vi "VNA_ReadConf.vi"(8 "error in":errorcluster, 10 "VNAClusterIn":T3={"Value"=0.0, "GUI Data Cluster"={"S11"=FALSE, "S21"=FALSE, "S12"=FALSE, "S22"=FALSE, "S11Meas"=enum."Log-magnitude (dB)", "S21Meas"=enum."Log-magnitude (dB)", "S12Meas"=enum."Log-magnitude (dB)", "S22Meas"=enum."Log-magnitude (dB)"}, "Timing"={"Last Operation"=0.0, "Stop @ T/B"=FALSE, "Last Temp"=0.0, "Last Mag"=0.0, "Ramp Param"={"End T (K)"=0.0, "Delta T (K)"=0.0, "End B (T)"=0.0, "Delta B (T)"=0.0}, "LastOp?"=FALSE, "FirstOp?"=FALSE}, "Measurements"=[], "Hardware"={"VNA TCP Con"=refnum, "VNA TCP Port"=5025, "Global T VAR"="", "Global B VAR"=""}, "Operation"={"Operation Mode"=enum."Logging", "Log Folder"=path "", "Measure Mode"=enum."Deltat"}}, 11 "GeneralClusterIn":T1) -> (0 "error out":errorcluster, 2 "VNAClusterOut":T3={"Value"=0.0, "GUI Data Cluster"={"S11"=FALSE, "S21"=FALSE, "S12"=FALSE, "S22"=FALSE, "S11Meas"=enum."Log-magnitude (dB)", "S21Meas"=enum."Log-magnitude (dB)", "S12Meas"=enum."Log-magnitude (dB)", "S22Meas"=enum."Log-magnitude (dB)"}, "Timing"={"Last Operation"=0.0, "Stop @ T/B"=FALSE, "Last Temp"=0.0, "Last Mag"=0.0, "Ramp Param"={"End T (K)"=0.0, "Delta T (K)"=0.0, "End B (T)"=0.0, "Delta B (T)"=0.0}, "LastOp?"=FALSE, "FirstOp?"=FALSE}, "Measurements"=[], "Hardware"={"VNA TCP Con"=refnum, "VNA TCP Port"=5025, "Global T VAR"="", "Global B VAR"=""}, "Operation"={"Operation Mode"=enum."Logging", "Log Folder"=path "", "Measure Mode"=enum."Deltat"}}, 3 "GeneralClusterOut":T1)   [LabVIEW 2021]
uses:
  Library/TerminalDef.ctl
  <vilib>/Utility/config.llb/Config Data RefNum.ctl
  Data_Cluster.ctl
  Measurement_Cluster.ctl
  Mode_Enum.ctl
  Library/LibDan.lvlib
  <vilib>/Utility/config.llb/NI_LVConfig.lvlib
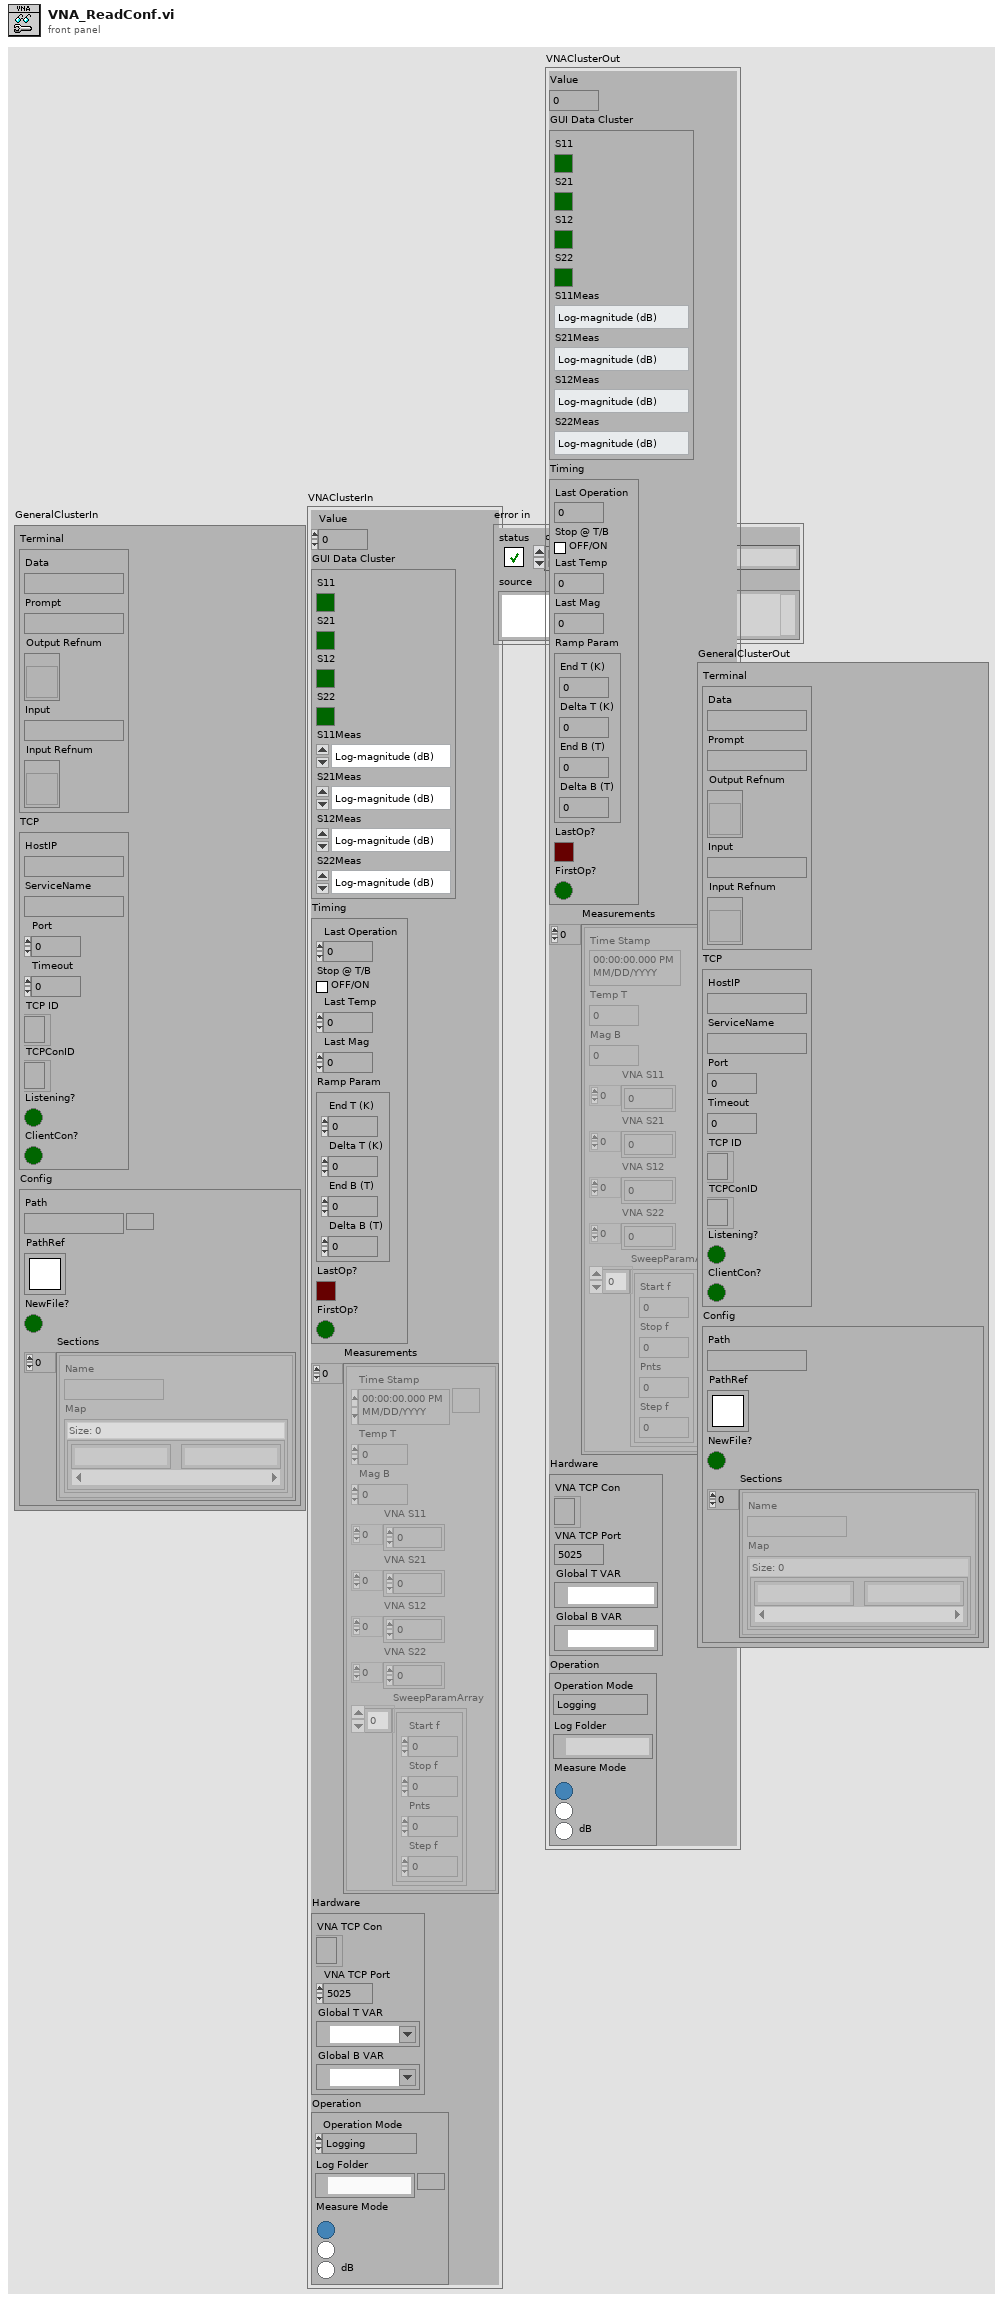
[diagram p1: front panel]
types:
  T1 = typedef "LibDan.lvlib/TerminalDef.ctl" = cluster{"Terminal":cluster{"Data":string, "Prompt":string, "Output Refnum":refnum<vi>, "Input":string, "Input Refnum":refnum<vi>}, "TCP":cluster{"HostIP":string, "ServiceName":string, "Port":u16, "Timeout":i32, "TCP ID":refnum<k5>, "TCPConID":refnum<k5>, "Listening?":bool, "ClientCon?":bool}, "Config":cluster{"Path":path, "PathRef":T2, "NewFile?":bool, "Sections":cluster{"Name":string, "Map":map{string, string}}[]}}
  T2 = typedef "NI_LVConfig.lvlib/Config Data RefNum.ctl" = refnum<k1>
  T3 = typedef "Data_Cluster.ctl" = cluster{"Value":dbl, "GUI Data Cluster":cluster{"S11":bool, "S21":bool, "S12":bool, "S22":bool, "S11Meas":enum16{"Log-magnitude (dB)", "Linear magnitude", "Phase (deg)", "Time Domain", "Real", "Imaginary", "Group Delay", "Polarlinear"}, "S21Meas":enum16{"Log-magnitude (dB)", "Linear magnitude", "Phase (deg)", "Time Domain", "Real", "Imaginary", "Group Delay", "Polarlinear"}, "S12Meas":enum16{"Log-magnitude (dB)", "Linear magnitude", "Phase (deg)", "Time Domain", "Real", "Imaginary", "Group Delay", "Polarlinear"}, "S22Meas":enum16{"Log-magnitude (dB)", "Linear magnitude", "Phase (deg)", "Time Domain", "Real", "Imaginary", "Group Delay", "Polarlinear"}}, "Timing":cluster{"Last Operation":dbl, "Stop @ T/B":bool, "Last Temp":dbl, "Last Mag":dbl, "Ramp Param":cluster{"End T (K)":dbl, "Delta T (K)":dbl, "End B (T)":dbl, "Delta B (T)":dbl}, "LastOp?":bool, "FirstOp?":bool}, "Measurements":T4[], "Hardware":cluster{"VNA TCP Con":refnum<k5>, "VNA TCP Port":i32, "Global T VAR":refnum<k21>, "Global B VAR":refnum<k21>}, "Operation":cluster{"Operation Mode":T5, "Log Folder":path, "Measure Mode":enum32{"Deltat", "DeltaT", "dB"}}}
  T4 = typedef "Measurement_Cluster.ctl" = cluster{"Time Stamp":timestamp, "Temp T":dbl, "Mag B":dbl, "VNA S11":dbl[], "VNA S21":dbl[], "VNA S12":dbl[], "VNA S22":dbl[], "SweepParamArray":cluster{"Start f":dbl, "Stop f":dbl, "Pnts":i32, "Step f":dbl}[]}
  T5 = typedef "Mode_Enum.ctl" = enum16{"Logging", "Idle-Off", "Idle"}
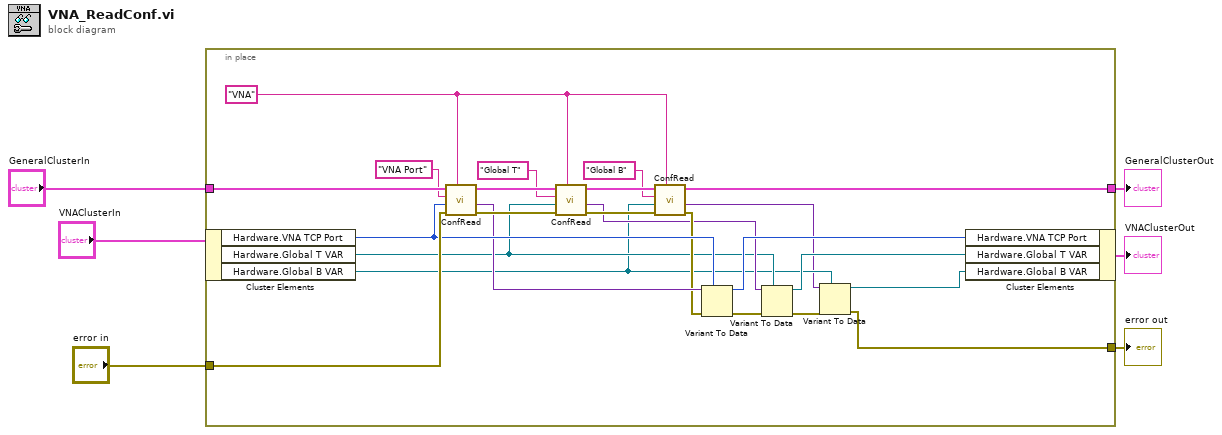
[diagram p0: block diagram]
diagram:
  n1 = in-place {
    in-place-border: "GeneralClusterIn" -> [w30]
    in-place-border: "error in" -> [w27]
    in-place-border: [w9] -> w1
    in-place-border: [w8] -> w3
    w10 = "VNA"
    n2 = in-place-cluster #1("VNAClusterIn") -> ("Hardware.VNA TCP Port"=w21:i32, "Hardware.Global T VAR"=w15:refnum<k21>, "Hardware.Global B VAR"=w12:refnum<k21>)
    n3 = call "ConfRead.vi"("Section"=w10, "error in"=w27, "type"=w21, "key"="VNA Port", "StructIn"=w30) -> ("error out"=w26:errorcluster, "value"=w20:variant, "StructOut"=w29:T1)  [unwired: 4 in]
    n4 = call "ConfRead.vi"("Section"=w10, "error in"=w26, "type"=w15, "key"="Global T", "StructIn"=w29) -> ("error out"=w23:errorcluster, "value"=w17:variant, "StructOut"=w24:T1)  [unwired: 4 in]
    n5 = call "ConfRead.vi"("Section"=w10, "error in"=w23, "type"=w12, "key"="Global B", "StructIn"=w24) -> ("error out"=w19:errorcluster, "value"=w11:variant, "StructOut"=w9:T1)  [unwired: 4 in]
    n6 = Variant To Data(error in=w19, type=w21, Variant=w20) -> (data=w18:i32, error out=w16:errorcluster)
    n7 = Variant To Data(error in=w16, type=w15, Variant=w17) -> (data=w14:refnum<k21>, error out=w13:errorcluster)
    n8 = Variant To Data(error in=w13, type=w12, Variant=w11) -> (data=w7:refnum<k21>, error out=w8:errorcluster)
    n9 = in-place-cluster #1("Hardware.VNA TCP Port"=w18, "Hardware.Global T VAR"=w14, "Hardware.Global B VAR"=w7) -> (→"VNAClusterOut":T3)
  }
  "error out" <- w3
  "GeneralClusterOut" <- w1
